vi "Check Transition.vi"(6 "Loop Data in":T1, 11 "Sequence in":refnum<class "Sequence.lvclass">) -> (4 "Loop Data":T1)   [LabVIEW 2023, in "VolatusSeq.lvlib" / "Sequence.lvclass"]
uses:
  Sequence.lvclass
  Loop Data.ctl
  Volatus/MessageQ/MessageQ.lvclass
  Sequence Time.ctl
  Sequence.lvclass/Sequence.ctl
  State/State.lvclass
  VolatusSeq.lvlib
  VolatusSeqConfig/Debug Flags.ctl
  VolatusSeqConfig/VolatusSeqConfig.lvlib
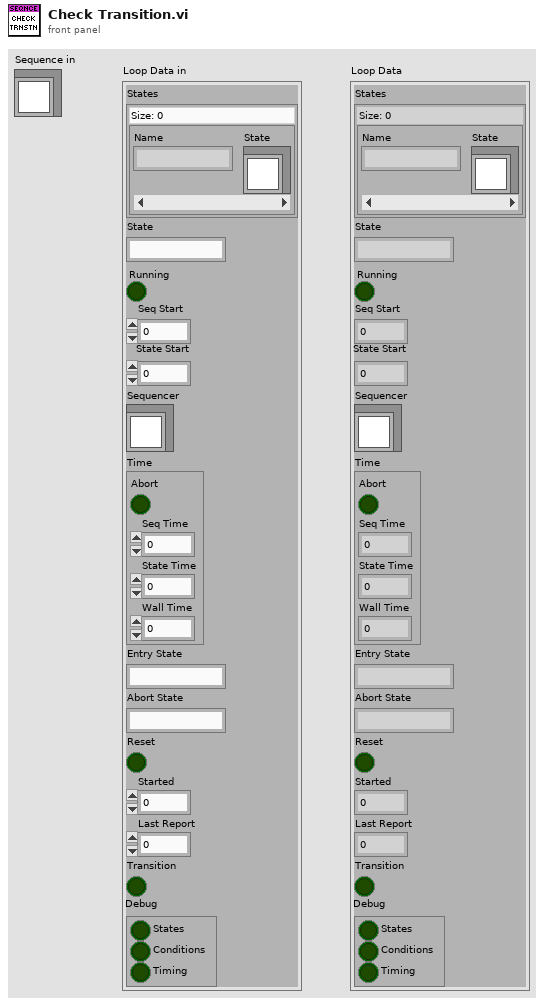
[diagram p1: front panel]
types:
  T1 = typedef "VolatusSeq.lvlib/Sequence.lvclass/Loop Data.ctl" = cluster{"States":map{string, refnum<class "State.lvclass">}, "State":string, "Running":bool, "Seq Start":dbl, "State Start":dbl, "Sequencer":refnum<class "MessageQ.lvclass">, "Time":T2, "Entry State":string, "Abort State":string, "Reset":bool, "Started":dbl, "Last Report":dbl, "Transition":bool, "Debug":T3}
  T2 = typedef "VolatusSeq.lvlib/Sequence Time.ctl" = cluster{"Abort":bool, "Seq Time":dbl, "State Time":dbl, "Wall Time":dbl}
  T3 = typedef "VolatusSeqConfig.lvlib/Debug Flags.ctl" = cluster{"States":bool, "Conditions":bool, "Timing":bool}
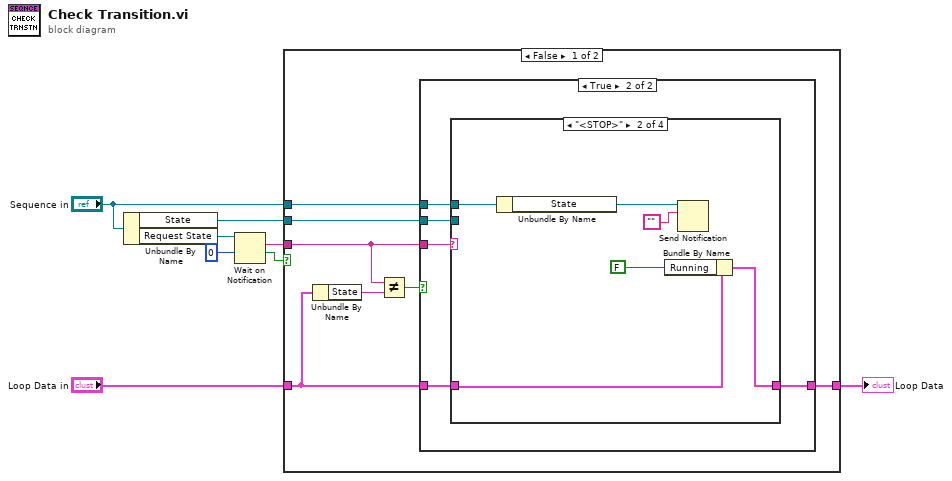
[diagram p0: block diagram]
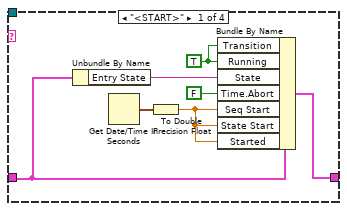
[diagram p3: hidden frame]
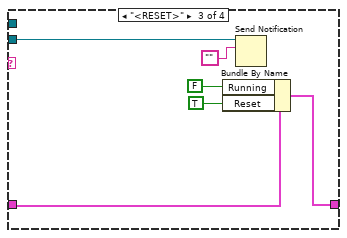
[diagram p4: hidden frame]
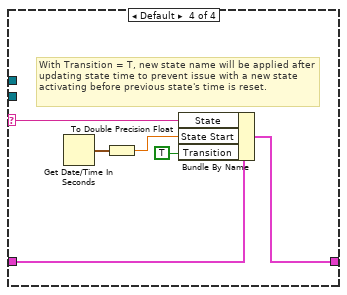
[diagram p5: hidden frame]
diagram:
  n1 = Unbundle By Name("Sequence in") -> ("State"=w1:refnum<notifier>, "Request State"=w8:refnum<notifier>)
  n2 = Wait on Notification(notifier=w8, timeout in ms (-1)=0) -> (notification=w5:string, timed out?=w6:bool)  [unwired: 2 in, 2 out]
  n3 = case shown="False" w6 {
    tunnel: w5 -> [w14 _]
    tunnel: "Loop Data in" -> [w11 w47]
    tunnel: [w13 w47] -> w3
    tunnel: "Sequence in" -> [w10 _]
    tunnel: w1 -> [w9 _]
    frame False {
      n4 = Unbundle By Name(w11) -> ("State"=w15:string)
      n5 = Not Equal?(x=w14, y=w15) -> (x != y?=w12:bool)
      n6 = case shown="True" w12 {
        tunnel: w11 -> [w16 w21]
        tunnel: w14 -> [_ w19]
        tunnel: [w16 w20] -> w13
        tunnel: w10 -> [_ w18]
        tunnel: w9 -> [_ w17]
        frame False {
        }
        frame True {
          n7 = case shown="\"<STOP>\"" w19 {
            selector: w19 -> [_ _ _ w42]
            tunnel: w21 -> [w25 w32 w38 w46]
            tunnel: [w27 w34 w40 w45] -> w20
            tunnel: w18 -> [_ w30 _ _]
            tunnel: w17 -> [_ _ w35 _]
            frame "<START>" {
              w22 = TRUE ("Running")
              n8 = Unbundle By Name(w25) -> ("Entry State"=w24:string)
              n9 = Get Date/Time In Seconds() -> (seconds since 1Jan1904=w28:timestamp)
              n10 = To Double Precision Float(number=w28) -> (double precision float=w23:dbl)
              n11 = Bundle By Name(cluster=w25, "Transition"=w22, "Running"=w22, "State"=w24, "Time.Abort"=FALSE ("Abort"), "Seq Start"=w23, "State Start"=w23, "Started"=w23) -> (w27:T1)
            }
            frame "<STOP>" {
              n12 = Unbundle By Name(w30) -> ("State"=w29:refnum<notifier>)
              n13 = Bundle By Name(cluster=w32, "Running"=FALSE) -> (w34:T1)
              n14 = Send Notification(notification="", notifier=w29) -> ()  [unwired: 1 in, 2 out]
            }
            frame "<RESET>" {
              n15 = Bundle By Name(cluster=w38, "Running"=FALSE, "Reset"=TRUE) -> (w40:T1)
              n16 = Send Notification(notification="", notifier=w35) -> ()  [unwired: 1 in, 2 out]
            }
            frame Default {
              # "With Transition = T, new state name will be applied after updating state time to prevent issue with a new state activating before previous state's time is reset."
              n17 = Get Date/Time In Seconds() -> (seconds since 1Jan1904=w44:timestamp)
              n18 = To Double Precision Float(number=w44) -> (double precision float=w43:dbl)
              n19 = Bundle By Name(cluster=w46, "State"=w42, "State Start"=w43, "Transition"=TRUE) -> (w45:T1)
            }
          }
        }
      }
    }
    frame True {
    }
  }
  "Loop Data" <- w3
